vi "随机数生成.vi"(11 "数组":dbl[](array[numeric])) -> (3 "簇":cluster{"行":i32, "列":i32})   [LabVIEW 2012]
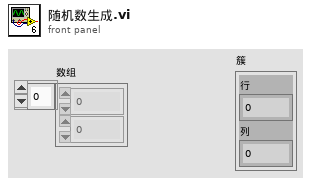
[diagram p1: front panel]
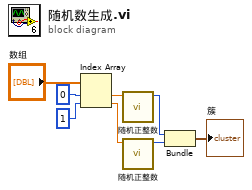
[diagram p0: block diagram]
diagram:
  n1 = Index Array(array="数组", index #1=0 ("索引"), index #2=1 ("索引")) -> (element #1=w3:dbl, element #2=w1:dbl)
  n2 = call "随机正整数.vi"("输入"=w3) -> ("输出"=w4:i32)  [unwired: 10 in]
  n3 = call "随机正整数.vi"("输入"=w1) -> ("输出"=w2:i32)  [unwired: 10 in]
  n4 = Bundle("输出"=w4, "输出"=w2) -> (→"簇":cluster{"输出":i32, "输出":i32})  [unwired: 1 in]
